vi "Initialize Popup.vi"(8 "error in (no error)":errorcluster, 9 "Size":T2, 10 "Screen Coordinates":T1, 11 "Path Data Type in":refnum<class "Path Data Type.lvclass">) -> (0 "error out":errorcluster, 2 "Dialog":refnum<class "Dialog.lvclass">, 3 "Path Data Type out":refnum<class "Path Data Type.lvclass">)   [LabVIEW 2018, in "Path Data Type.lvclass"]
uses:
  Path Data Type.lvclass
  <vilib>/MGI/Panel Manager/Panel/Panel/Window/Dialog/Dialog.lvclass
  <vilib>/Utility/miscctls.llb/LVBoundsTypeDef.ctl
  <vilib>/Utility/miscctls.llb/LVPointTypeDef.ctl
  <vilib>/MGI/Panel Manager/Panel/Panel/Window/Dialog/Behavior.ctl
  <vilib>/MGI/Panel Manager/Panel/Window Position/Reference Position/Size/Absolute Size/Absolute Size.lvclass/Absolute Size.ctl
  <vilib>/MGI/Panel Manager/Panel/Window Position/Reference Position/Offset/Absolute Offset/Absolute Offset.lvclass/Absolute Offset.ctl
  <vilib>/MGI/Panel Manager/Panel/Window Position/Reference Position/Size/Absolute Size/Absolute Size.vi
  <vilib>/MGI/Panel Manager/Panel/Window Position/Reference Position/Offset/Absolute Offset/Absolute Offset.vi
  <vilib>/MGI/Panel Manager/Panel/Window Position/Reference Position/Size/Absolute Size/Absolute Size.lvclass
  C:/Program Files (x86)/National Instruments/LabVIEW 2018/vi.lib/MGI/Panel Manager/Panel/Window Position/Reference Position/Size/Size.lvclass
  <vilib>/MGI/Panel Manager/Panel/Window Position/Reference Position/Offset/Absolute Offset/Absolute Offset.lvclass
  C:/Program Files (x86)/National Instruments/LabVIEW 2018/vi.lib/MGI/Panel Manager/Panel/Window Position/Reference Position/Offset/Offset.lvclass
  <vilib>/MGI/Panel Manager/Panel/Window Position/Reference Position/Ref Display/Ref Display.lvclass
  C:/Program Files (x86)/National Instruments/LabVIEW 2018/vi.lib/MGI/Panel Manager/Panel/Window Position/Window Position.lvclass
  <vilib>/MGI/Panel Manager/Panel/Window Position/Reference Position/Ref Display/Ref Display.vi
  <vilib>/MGI/Panel Manager/Panel/Panel/Window/Dialog/Dialog.vi
  <vilib>/MGI/Panel Manager/Panel/Panel.lvlib
  C:/Program Files (x86)/National Instruments/LabVIEW 2018/vi.lib/MGI/Panel Manager/Panel/Window Position/Reference Position/Reference Position.lvclass
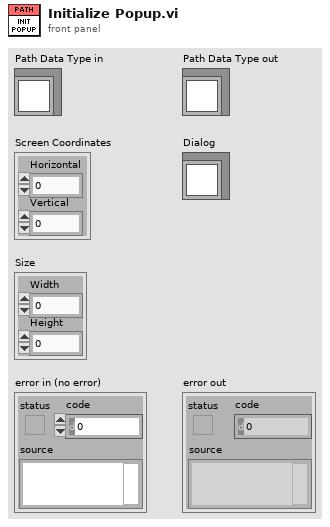
[diagram p1: front panel]
types:
  T1 = typedef "LVPointTypeDef.ctl" = cluster{"Horizontal":i16, "Vertical":i16}
  T2 = typedef "LVBoundsTypeDef.ctl" = cluster{"Width":u32, "Height":u32}
  T3 = typedef "Panel.lvlib/Dialog.lvclass/Behavior.ctl" = enum32{"Floating", "Floating/Auto-Hide", "Modal"}
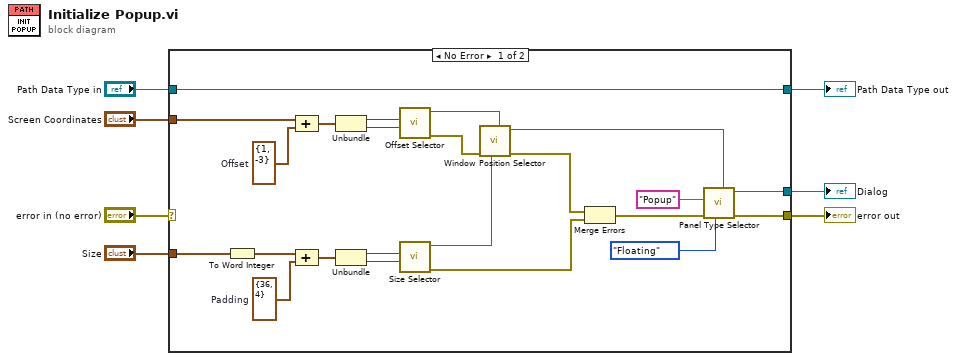
[diagram p0: block diagram]
diagram:
  n1 = case shown="No Error" "error in (no error)" {
    selector: "error in (no error)" -> [_ w32]
    tunnel: [w11 w32] -> w3
    tunnel: [w10 w31] -> w1
    tunnel: "Path Data Type in" -> [w10 w31]
    tunnel: [w16 _] -> w2
    tunnel: "Screen Coordinates" -> [w9 _]
    tunnel: "Size" -> [w8 _]
    frame No Error {
      w29 = cluster{"Width":i16, "Height":i16} {"Width"=1, "Height"=-3}  # Offset
      w25 = cluster{"Width":i16, "Height":i16} {"Width"=36, "Height"=4}  # Padding
      n2 = To Word Integer(number=w8) -> (16bit integer=w23:cluster{"Width":i16, "Height":i16})
      n3 = Compound Arithmetic op=ADD(w9, w29) -> (w28:T1)
      n4 = Compound Arithmetic op=ADD(w23, w25) -> (w24:cluster{"Width":i16, "Height":i16})
      n5 = Unbundle(w28) -> ("Horizontal"=w26:i16, "Vertical"=w27:i16)
      n6 = Unbundle(w24) -> ("Width"=w21:i16, "Height"=w22:i16)
      n7 = call-poly <vilib>:"Offset Selector.vi"("Vertical"=w27, "Horizontal"=w26) -> ("Error Out"=w15:errorcluster, "Absolute Offset Out"=w20:refnum<class "Absolute Offset.lvclass">)  [unwired: 8 in]
      n8 = call-poly <vilib>:"Size Selector.vi"("Height"=w22, "Width"=w21) -> ("Error Out"=w12:errorcluster, "Absolute Size out"=w19:refnum<class "Absolute Size.lvclass">)  [unwired: 8 in]
      n9 = call-poly <vilib>:"Window Position Selector.vi"("Offset"=w20, "Size"=w19, "Error In"=w15) -> ("Error Out"=w13:errorcluster, "Ref Display out"=w18:refnum<class "Ref Display.lvclass">)  [unwired: 7 in]
      n10 = Merge Errors(w13, w12) -> (w14:errorcluster)
      n11 = call-poly <vilib>:"Panel Type Selector.vi"("Window Position (Center in Top Level)"=w18, "Behavior (Modal)"=Behavior."Floating", "Error In"=w14, "Default Title"="Popup") -> ("Error Out"=w11:errorcluster, "Dialog out"=w16:refnum<class "Dialog.lvclass">)  [unwired: 6 in]
    }
    frame Error {
    }
  }
  "error out" <- w3
  "Path Data Type out" <- w1
  "Dialog" <- w2
